vi "RM.treeTagToFilter.vi"(11 "tree tag":string) -> (3 "filter type":i32)   [LabVIEW 2016, in "FPGA Resource Manager.lvlib"]
uses:
  FPGA Resource Manager.lvlib
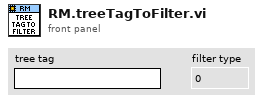
[diagram p1: front panel]
types:
  T1 = typedef "FPGA Resource Manager.lvlib/RM.resourceType.ctl" = enum16{"Scalar Input", "Scalar Output", "Waveform Input", "Waveform Output"}
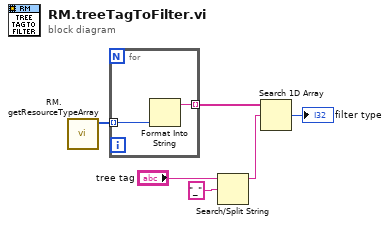
[diagram p0: block diagram]
diagram:
  n1 = call "RM.getResourceTypeArray.vi"() -> ("Array"=w5:T1[])  [unwired: 11 in]
  n2 = for {
    tunnel: w5 -> [w8] mode=indexing
    tunnel: [w7] -> w6 mode=indexing
    n3 = Format Into String(w8) -> (resulting string=w7:string)  [unwired: 3 in, 1 out]
  }
  n4 = Search/Split String(string="tree tag", search string/char (-)="_") -> (substring before match=w1:string)  [unwired: 1 in, 2 out]
  n5 = Search 1D Array(1D array=w6, element=w1) -> (index of element=→"filter type":i32)  [unwired: 1 in]
